vi "simple histograms.vi"(0 "Host Plot Controls":T2={"refresh"=FALSE, "PMTs for Host"={"Sa"=1, "Sb"=0, "g-factor"=1}, "Peaks"={"# bins"=100, "min"=0.0, "max"=10.0}, "Averages"={"# bins"=100, "max"=10.0, "min"=0.0}, "Durations"={"# bins"=100, "max"=10.0, "min"=0.0}, "FP-FPGA"={"# bins"=100, "max"=50.0, "min"=0.0}, "FP-Host"={"# bins"=100, "max"=12.0, "min"=8.0}}, 4 "peaks data":T1) -> (16 "Number of drops detected":i32, 20 "H(average) vs average [volts]":cluster{"Axis":dbl[], i32[]}[](graph), 21 "H(peaks) vs peaks [volts]":cluster{"Axis":dbl[], i32[]}[](graph), 22 "H(durations) vs. durations [ms]":cluster{"Axis":dbl[], i32[]}(graph), 23 "FPGA_H(FP) vs. FP":cluster{"Axis":dbl[], i32[]}(graph), 27 "?":T3)   [LabVIEW 2009]
uses:
  <vilib>/Analysis/NI_AALPro.lvlib
  <vilib>/Analysis/NI_AALBase.lvlib
panel:
  out "H(durations) vs. durations [ms] 2":cluster{"Axis":dbl[], i32[]}(graph)
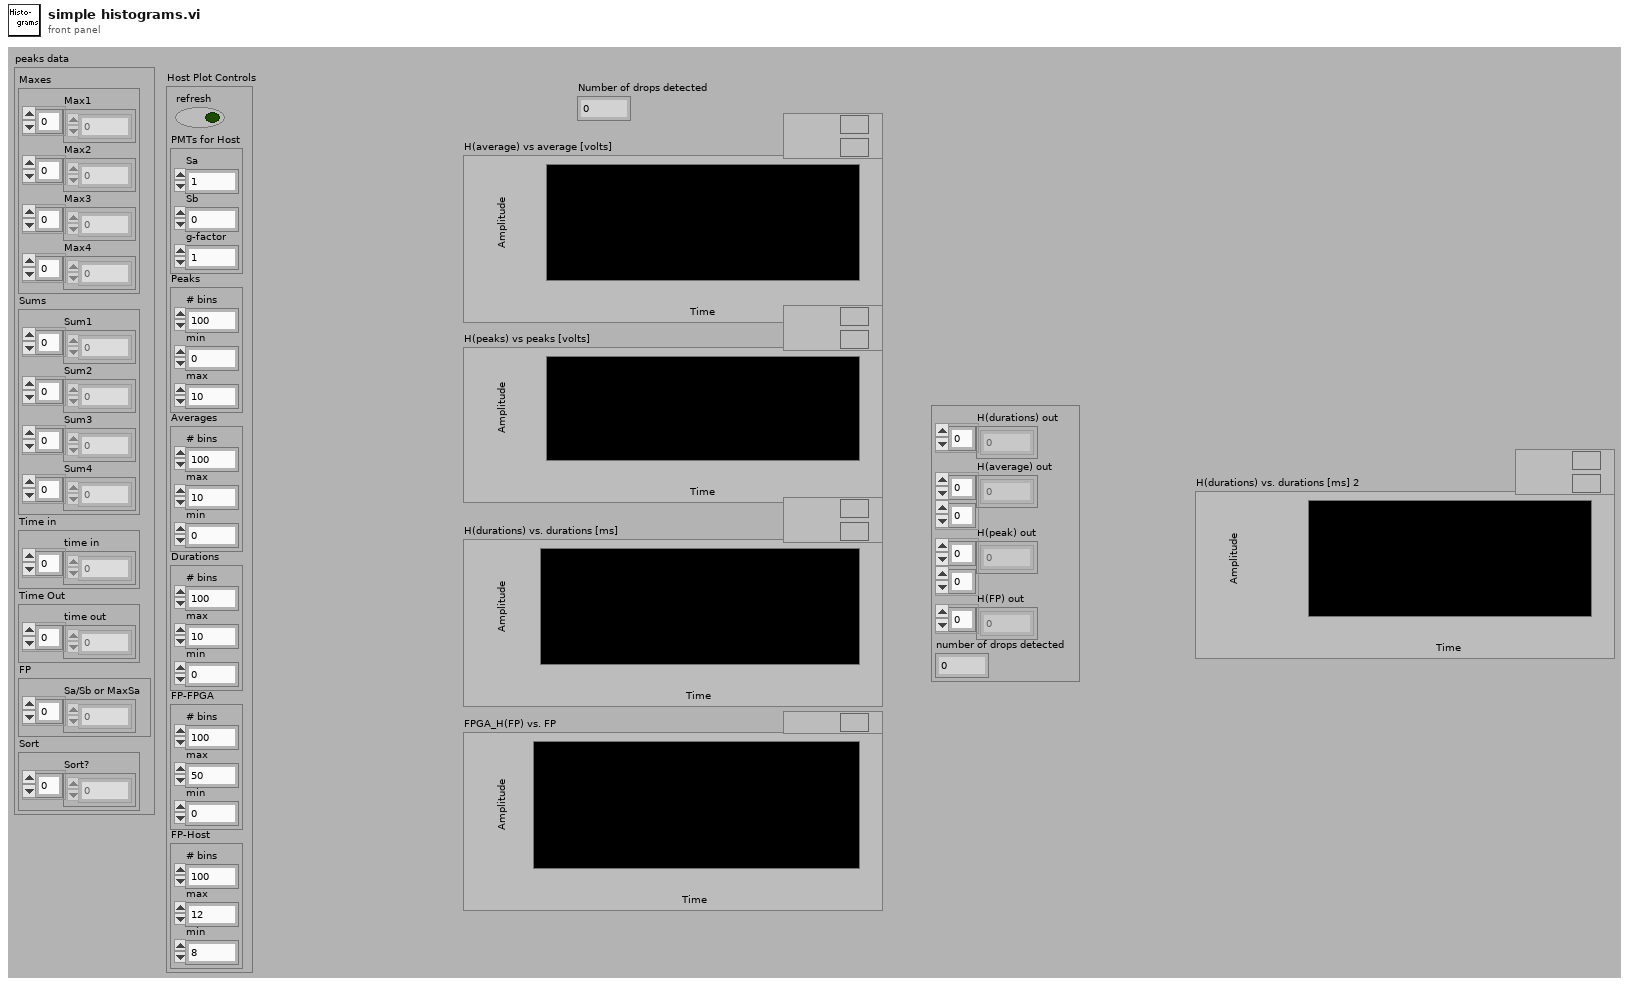
[diagram p1: front panel]
types:
  T1 = cluster{"Maxes":cluster{"Max1":dbl[], "Max2":dbl[], "Max3":dbl[], "Max4":dbl[]}, "Sums":cluster{"Sum1":dbl[], "Sum2":dbl[], "Sum3":dbl[], "Sum4":dbl[]}, "Time in":cluster{"time in":dbl[]}, "Time Out":cluster{"time out":dbl[]}, "FP":cluster{"Sa/Sb or MaxSa":dbl[]}, "Sort":cluster{"Sort?":dbl[]}}
  T2 = cluster{"refresh":bool, "PMTs for Host":cluster{"Sa":i8, "Sb":i8, "g-factor":i32}, "Peaks":cluster{"# bins":i32, "min":dbl, "max":dbl}, "Averages":cluster{"# bins":i32, "max":dbl, "min":dbl}, "Durations":cluster{"# bins":i32, "max":dbl, "min":dbl}, "FP-FPGA":cluster{"# bins":i32, "max":dbl, "min":dbl}, "FP-Host":cluster{"# bins":i32, "max":dbl, "min":dbl}}
  T3 = cluster{"H(durations) out":i32[], "H(average) out":i32[][], "H(peak) out":i32[][], "H(FP) out":i32[], "number of drops detected":i32}
  T4 = cluster{"Sum1":dbl[], "Sum2":dbl[], "Sum3":dbl[], "Sum4":dbl[]}
  T5 = cluster{"X Values":dbl[], "Histogram: h(x)":i32[]}
  T6 = cluster{"X Values":dbl[], "H(average) out":i32[]}
  T7 = cluster{"H(durations) out":i32[], "H(average) out":i32[][], "H(average) out":i32[][], "H(FP) out":i32[], i32}
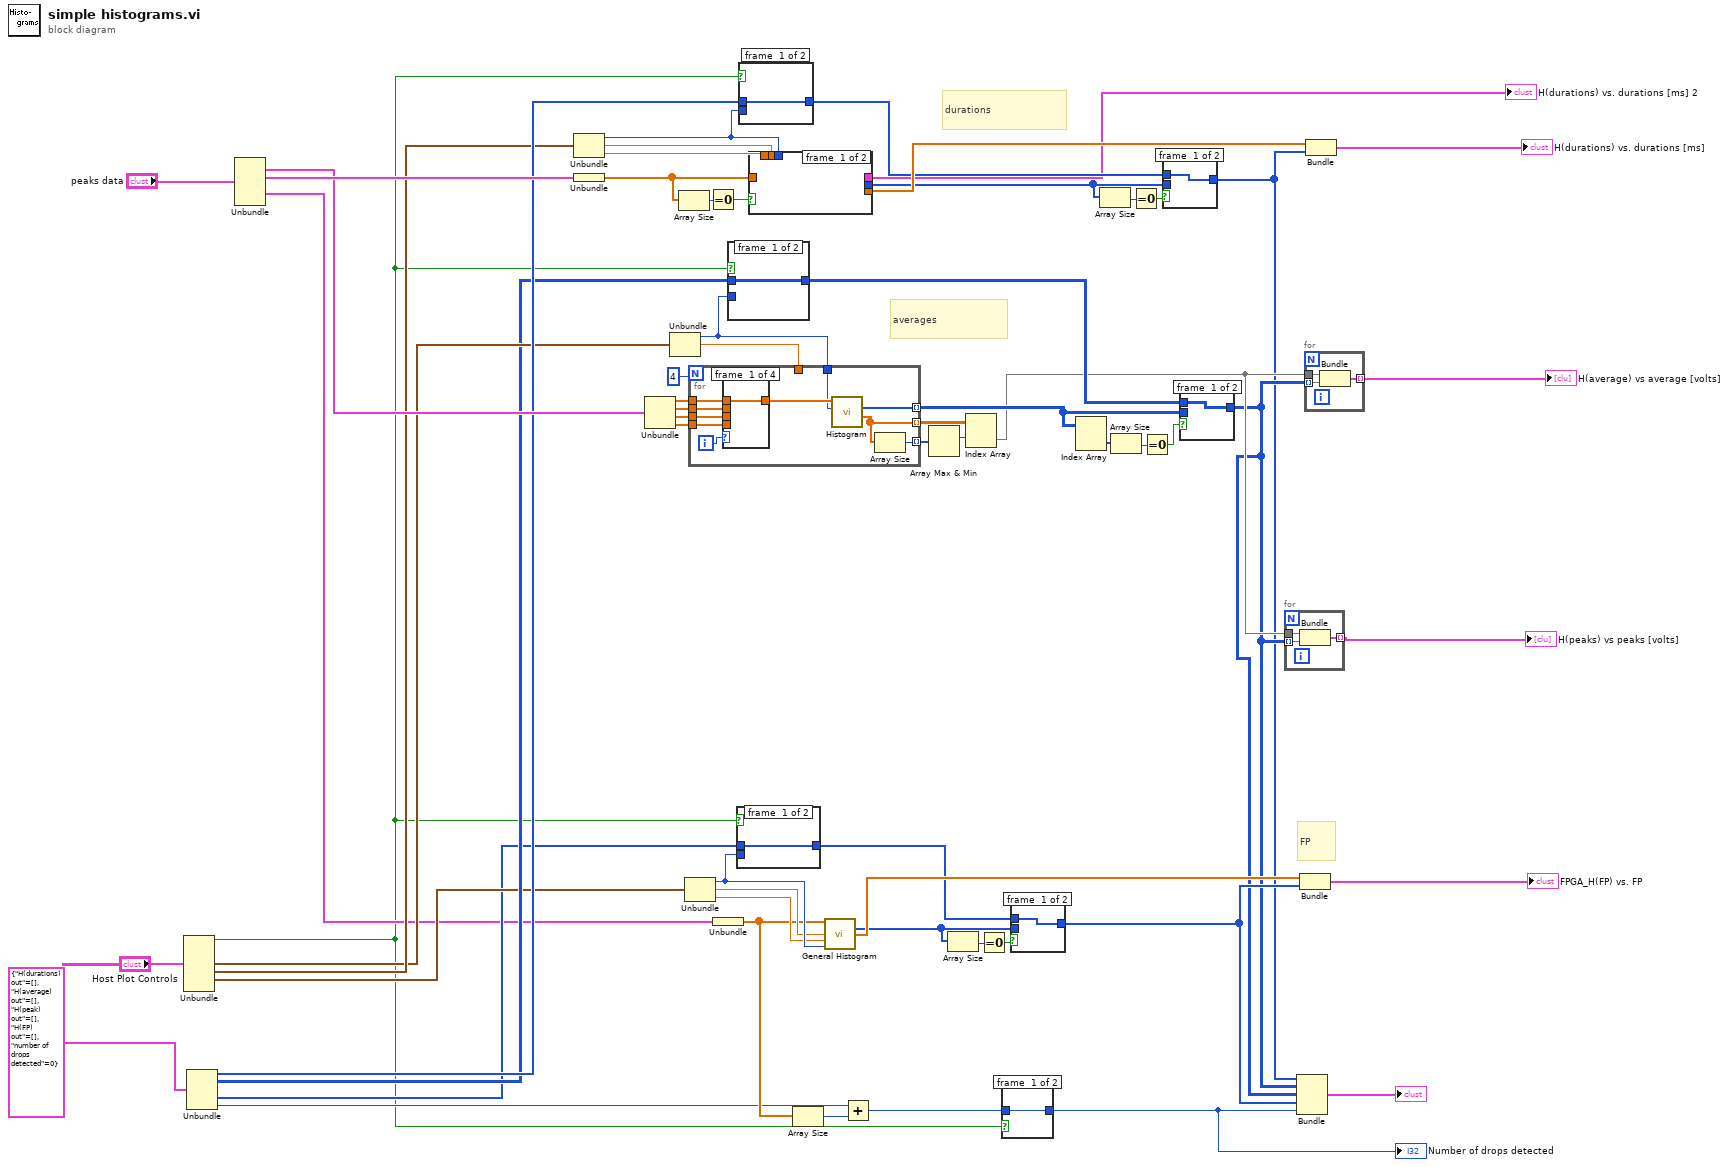
[diagram p0: block diagram]
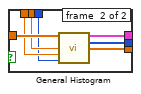
[diagram p2: hidden frame]
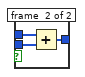
[diagram p3: hidden frame]
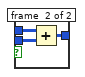
[diagram p4: hidden frame]
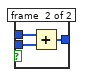
[diagram p5: hidden frame]
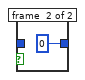
[diagram p6: hidden frame]
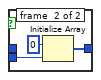
[diagram p7: hidden frame]
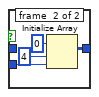
[diagram p8: hidden frame]
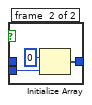
[diagram p9: hidden frame]
diagram:
  # "durations"
  # "averages"
  # "FP"
  n1 = Unbundle("Host Plot Controls") -> ("refresh"=w26:bool, "Averages"=w40:cluster{"# bins":i32, "max":dbl, "min":dbl}, "Durations"=w41:cluster{"# bins":i32, "max":dbl, "min":dbl}, "FP-FPGA"=w31:cluster{"# bins":i32, "max":dbl, "min":dbl})  [unwired: 3 out]
  n2 = Unbundle(T3 {"H(durations) out"=[], "H(average) out"=[], "H(peak) out"=[], "H(FP) out"=[], "number of drops detected"=0}) -> ("H(durations) out"=w42:i32[], "H(average) out"=w37:i32[][], "H(FP) out"=w30:i32[], "number of drops detected"=w27:i32)  [unwired: 1 out]
  n3 = Unbundle("peaks data") -> ("Sums"=w47:T4, "Time in"=w48:cluster{"time in":dbl[]}, "FP"=w29:cluster{"Sa/Sb or MaxSa":dbl[]})  [unwired: 3 out]
  n4 = Unbundle(w41) -> ("# bins"=w44:i32, "max"=w46:dbl, "min"=w45:dbl)
  n5 = Unbundle(w48) -> ("time in"=w3:dbl[])
  n6 = Unbundle(w47) -> ("Sum1"=w49:dbl[], "Sum2"=w50:dbl[], "Sum3"=w51:dbl[], "Sum4"=w52:dbl[])
  n7 = Unbundle(w40) -> ("# bins"=w38:i32, "max"=w39:dbl)  [unwired: 1 out]
  n8 = Array Size(array=w3) -> (size(s)=w2:i32)
  n9 = Unbundle(w31) -> ("# bins"=w35:i32, "max"=w33:dbl, "min"=w34:dbl)
  n10 = for {
    N: 4 -> [_]
    tunnel: w49 -> [w71]
    tunnel: w50 -> [w70]
    tunnel: w51 -> [w69]
    tunnel: w52 -> [w68]
    tunnel: [w67] -> w15 mode=indexing
    tunnel: [w66] -> w54 mode=indexing
    tunnel: [w65] -> w55 mode=indexing
    tunnel: w39 -> [_]
    tunnel: w38 -> [w63]
    i -> [w72]
    n11 = case shown="3" w72 {
      tunnel: w71 -> [w73 _ _ _]
      tunnel: w70 -> [_ w74 _ _]
      tunnel: w69 -> [_ _ w75 _]
      tunnel: w68 -> [_ _ _ w76]
      tunnel: [w73 w74 w75 w76] -> w64
      frame #0 {
      }
      frame #1 {
      }
      frame #2 {
      }
      frame #3 {
      }
    }
    n12 = call <vilib>:"Histogram.vi"("intervals"=w63, "X"=w64) -> ("X Values"=w65:dbl[], "Histogram: h(x)"=w67:i32[])  [unwired: 6 in, 2 out]
    n13 = Array Size(array=w65) -> (size(s)=w66:i32)
  }
  n14 = Equal To 0?(x=w2) -> (x = 0?=w1:bool)
  n15 = Unbundle(w29) -> ("Sa/Sb or MaxSa"=w28:dbl[])
  n16 = case shown="True" w26 {
    tunnel: [w77 w80] -> w17
    tunnel: w38 -> [_ w79]
    tunnel: w37 -> [w77 _]
    frame #0 {
    }
    frame #1 {
      n17 = Initialize Array(0, 4, w79) -> (w80:i32[][])
    }
  }
  n18 = case shown="True" w26 {
    tunnel: [w82 w84] -> w12
    tunnel: w35 -> [_ w83]
    tunnel: w30 -> [w82 _]
    frame #0 {
    }
    frame #1 {
      n19 = Initialize Array(0, w83) -> (w84:i32[])
    }
  }
  n20 = case shown="True" w26 {
    tunnel: [w86 w88] -> w43
    tunnel: w44 -> [_ w87]
    tunnel: w42 -> [w86 _]
    frame #0 {
    }
    frame #1 {
      n21 = Initialize Array(0, w87) -> (w88:i32[])
    }
  }
  n22 = case shown="True" w1 {
    tunnel: [_ w96] -> w61
    tunnel: w3 -> [_ w95]
    tunnel: w46 -> [_ w94]
    tunnel: w45 -> [_ w93]
    tunnel: w44 -> [_ w92]
    tunnel: [_ w91] -> w22
    tunnel: [_ w90] -> w4
    frame #0 {
    }
    frame #1 {
      n23 = call <vilib>:"General Histogram.vi"("X"=w95, "max"=w94, "min"=w93, "# bins"=w92) -> ("Histogram Graph"=w90:T5, "Histogram"=w91:i32[], "Axis"=w96:dbl[])  [unwired: 7 in, 2 out]
    }
  }
  "H(durations) vs. durations [ms] 2" <- w4
  n24 = Array Size(array=w28) -> (size(s)=w58:i32)
  n25 = call <vilib>:"General Histogram.vi"("X"=w28, "max"=w33, "min"=w34, "# bins"=w35) -> ("Histogram"=w11:i32[], "Axis"=w32:dbl[])  [unwired: 7 in, 3 out]
  n26 = Add(x=w27, y=w58) -> (x+y=w25:i32)
  n27 = Array Max & Min(array=w54) -> (max index (indices)=w56:i32)  [unwired: 3 out]
  n28 = Array Size(array=w11) -> (size(s)=w13:i32)
  n29 = Index Array(array=w55, index (row)=w56) -> (element=w7:dbl[])  [unwired: 1 in]
  n30 = Equal To 0?(x=w13) -> (x = 0?=w14:bool)
  n31 = case shown="True" w26 {
    tunnel: w25 -> [w97 _]
    tunnel: [w97 0] -> w24
    frame #0 {
    }
    frame #1 {
    }
  }
  "Number of drops detected" <- w24
  n32 = case shown="False" w14 {
    tunnel: [w99 w102] -> w10
    tunnel: w12 -> [w99 w101]
    tunnel: w11 -> [_ w100]
    frame #0 {
    }
    frame #1 {
      n33 = Add(x=w101, y=w100) -> (x+y=w102:i32[])
    }
  }
  n34 = Index Array(array=w15) -> (element=w16:i32[])  [unwired: 2 in]
  n35 = Array Size(array=w22) -> (size(s)=w21:i32)
  n36 = Array Size(array=w16) -> (size(s)=w18:i32)
  n37 = Equal To 0?(x=w21) -> (x = 0?=w20:bool)
  n38 = Equal To 0?(x=w18) -> (x = 0?=w19:bool)
  n39 = case shown="True" w20 {
    tunnel: [w103 w106] -> w5
    tunnel: w43 -> [w103 w105]
    tunnel: w22 -> [_ w104]
    frame #0 {
    }
    frame #1 {
      n40 = Add(x=w105, y=w104) -> (x+y=w106:i32[])
    }
  }
  n41 = case shown="False" w19 {
    tunnel: [w107 w110] -> w6
    tunnel: w17 -> [w107 w109]
    tunnel: w15 -> [_ w108]
    frame #0 {
    }
    frame #1 {
      n42 = Add(x=w109, y=w108) -> (x+y=w110:i32[][])
    }
  }
  n43 = for {
    tunnel: w7 -> [w113]
    tunnel: w6 -> [w112] mode=indexing
    tunnel: [w111] -> w36 mode=indexing
    n44 = Bundle("X Values"=w113, "H(average) out"=w112) -> (w111:T6)  [unwired: 1 in]
  }
  "H(peaks) vs peaks [volts]" <- w36
  n45 = Bundle("H(durations) out"=w5, "H(average) out"=w6, "H(average) out"=w6, "H(FP) out"=w10, w24) -> (→"?":T7)  [unwired: 1 in]
  n46 = Bundle("Axis"=w32, "H(FP) out"=w10) -> (→"FPGA_H(FP) vs. FP":cluster{"Axis":dbl[], "H(FP) out":i32[]})  [unwired: 1 in]
  n47 = for {
    tunnel: w7 -> [w116]
    tunnel: w6 -> [w115] mode=indexing
    tunnel: [w114] -> w62 mode=indexing
    n48 = Bundle("X Values"=w116, "H(average) out"=w115) -> (w114:T6)  [unwired: 1 in]
  }
  "H(average) vs average [volts]" <- w62
  n49 = Bundle("Axis"=w61, "H(durations) out"=w5) -> (→"H(durations) vs. durations [ms]":cluster{"Axis":dbl[], "H(durations) out":i32[]})  [unwired: 1 in]
